vi "Clear-object.vi"(8 "error in (no error)":errorcluster, 11 "Object ref in":T1) -> (0 "error out":errorcluster)   [LabVIEW 2013, in "PowderDeposition.lvlib" / "PD-Main.lvclass"]
uses:
  PD-Main.lvclass
  Object-reference.ctl
  Client-status.ctl
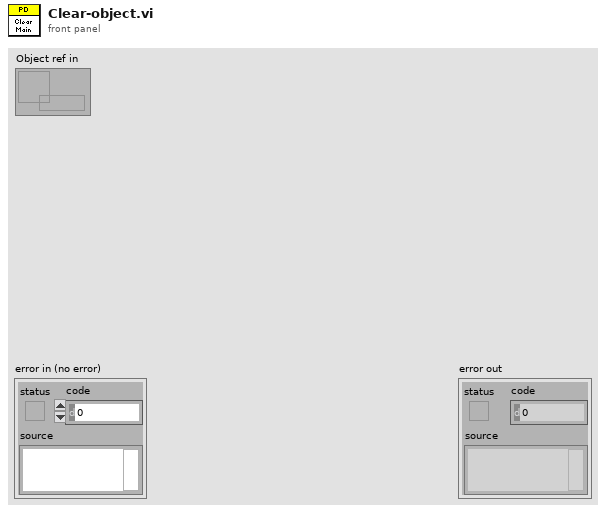
[diagram p1: front panel]
types:
  T1 = typedef "PowderDeposition.lvlib/PD-Main.lvclass/Object-reference.ctl" = refnum<data-value>
  T2 = typedef "PowderDeposition.lvlib/PD-Main.lvclass/Client-status.ctl" = enum16{"Idle", "Initialized", "Configured", "Activated", "Started", "Paused", "Stopped", "Reset", "Error", "Exited"}
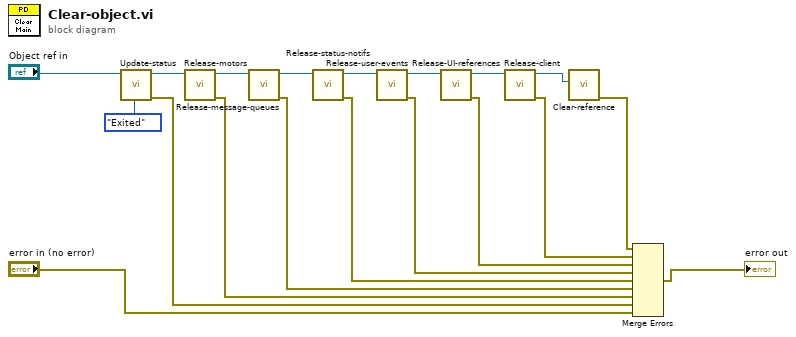
[diagram p0: block diagram]
diagram:
  n1 = call "Update-status.vi"("Status"=Client-status."Exited", "Object ref in"="Object ref in") -> ("error out"=w1:errorcluster, "Object ref out"=w2:T1)  [unwired: 8 in]
  n2 = call "Release-motors.vi"("Object ref in"=w2) -> ("error out"=w5:errorcluster, "Object ref out"=w7:T1)  [unwired: 9 in]
  n3 = call "Release-message-queues.vi"("Object ref in"=w7) -> ("error out"=w14:errorcluster, "Object ref out"=w18:T1)  [unwired: 9 in]
  n4 = call "Release-status-notifs.vi"("Object ref in"=w18) -> ("error out"=w13:errorcluster, "Object ref out"=w17:T1)  [unwired: 9 in]
  n5 = call "Release-user-events.vi"("Object ref in"=w17) -> ("error out"=w12:errorcluster, "Object ref out"=w11:T1)  [unwired: 9 in]
  n6 = call "Release-UI-references.vi"("Object ref in"=w11) -> ("error out"=w8:errorcluster, "Object ref out"=w10:T1)  [unwired: 9 in]
  n7 = call "Release-client.vi"("Object ref in"=w10) -> ("error out"=w9:errorcluster, "Object ref out"=w6:T1)  [unwired: 9 in]
  n8 = call "Clear-reference.vi"("Data ref"=w6) -> ("error out"=w16:errorcluster)  [unwired: 10 in]
  n9 = Merge Errors(w16, w9, w8, w12, w13, w14, w5, w1, "error in (no error)") -> (→"error out":errorcluster)
